vi "Create Dataset 3D Integer.vi"(7 "Chunk size":u64, 8 "error in (no error)":errorcluster, 9 "Datatype":i32[][][](array[numeric]), 10 "Dataset name":string, 11 "loc_id":i32) -> (0 "error out":errorcluster, 3 "Dataset id":i32)   [LabVIEW 2014]
uses:
  Release/HDF5Tools.dll
  HDF5Tools.lvlib
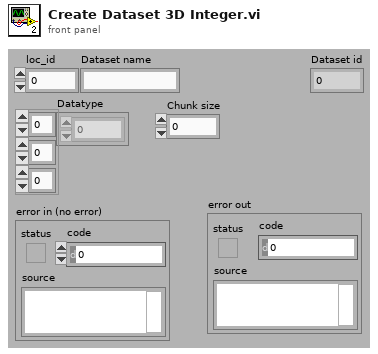
[diagram p1: front panel]
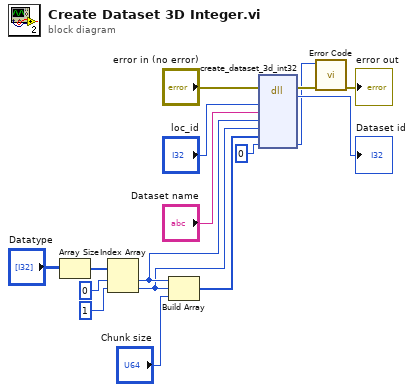
[diagram p0: block diagram]
diagram:
  n1 = Array Size(array="Datatype") -> (size(s)=w9:i32[])
  n2 = Index Array(array=w9, index #1=0 ("index"), index #2=1 ("index")) -> (element #1=w5:i32, element #2=w4:i32)
  n3 = Build Array(w5, w4, "Chunk size") -> (w3:u64[])
  n4 = dll-call lib="C:/HDF5Tools/Release/HDF5Tools.dll" fn="create_dataset_3d_int32"(error in="error in (no error)", "loc_id"="loc_id", "name"="Dataset name", "dim1"=w5, "dim2"=w4, "chunks"=w3, "error"=0) -> (error out=w12:errorcluster, "dataset_id"=→"Dataset id":i32, "error"=w10:i32)  [unwired: 7 in, 1 out]
  n5 = call "Error Code.vi"("Error in"=w12, "Error code"=w10) -> ("Error out"=→"error out":errorcluster)  [unwired: 9 in]
